vi "Configure Trigger Synchronization.vi"(0 "niUsrpRio Session":T1={"Global Settings Register Bus"=refnum, "Radio 0 Settings Register Bus"=refnum, "Rx NI-USRP session"="", "Tx NI-USRP session"="", "FPGA Interface"=refnum, "RIO Interface Number"=0, "EEPROM Header"={"Checksum"=0, "Product Code"=0, "Hardware Current Version"=0, "Hardware Oldest Compatible Version"=0, "EEPROM Map Current Version"=0, "EEPROM Map Oldest Compatible Version"=0, "User Password"="", "Pointer to Factory Header"=0, "Pointer to User Header"=0, "Recommended Interval"=0, "Number of Reserved Bytes"=9, "Number of Daughterboards"=0, "Daughterboard IDs"=[], "Daughterboard Serial Numbers"=[]}, "Device Data Header"={"Checksum"=0, "Number of Channels"=0, "Number of Gain Settings"=[], "Pointer to Characterization Data"=[], "Number of Reserved Bytes"=27, "Number of Frequencies"=[]}, "EEPROM Characterization Header"={"Checksum"=0, "Date"=timestamp(0 s since 1904-01-01), "Temperature"=0.0, "Misc. Info"="", "Pointer to Device Data Header"=0, "Number of Reserved Bytes"=28}, "Characterization Data"=[], "Characterization Data Valid?"=FALSE, "Radio 1 Settings Register Bus"=refnum, "Radio Settings Bus Semaphore"=refnum} {"Characterization Data"."Frequencies [Hz]" format="%#_6p"; "EEPROM Characterization Header"."Pointer to Device Data Header" format="%x"; "EEPROM Characterization Header"."Checksum" format="%x"; "Device Data Header"."Pointer to Characterization Data" format="%x"; "Device Data Header"."Checksum" format="%x"; "EEPROM Header"."Pointer to User Header" format="%x"; "EEPROM Header"."Pointer to Factory Header" format="%x"; "EEPROM Header"."Product Code" format="%x"; "EEPROM Header"."Checksum" format="%x"}, 1 "scope":string(combo)="rx", 5 "enable trigger synchronization":bool, 11 "error in":errorcluster) -> (4 "niUsrpRio Session (out)":T1={"Global Settings Register Bus"=refnum, "Radio 0 Settings Register Bus"=refnum, "Rx NI-USRP session"="", "Tx NI-USRP session"="", "FPGA Interface"=refnum, "RIO Interface Number"=0, "EEPROM Header"={"Checksum"=0, "Product Code"=0, "Hardware Current Version"=0, "Hardware Oldest Compatible Version"=0, "EEPROM Map Current Version"=0, "EEPROM Map Oldest Compatible Version"=0, "User Password"="", "Pointer to Factory Header"=0, "Pointer to User Header"=0, "Recommended Interval"=0, "Number of Reserved Bytes"=9, "Number of Daughterboards"=0, "Daughterboard IDs"=[], "Daughterboard Serial Numbers"=[]}, "Device Data Header"={"Checksum"=0, "Number of Channels"=0, "Number of Gain Settings"=[], "Pointer to Characterization Data"=[], "Number of Reserved Bytes"=27, "Number of Frequencies"=[]}, "EEPROM Characterization Header"={"Checksum"=0, "Date"=timestamp(0 s since 1904-01-01), "Temperature"=0.0, "Misc. Info"="", "Pointer to Device Data Header"=0, "Number of Reserved Bytes"=28}, "Characterization Data"=[], "Characterization Data Valid?"=FALSE, "Radio 1 Settings Register Bus"=refnum, "Radio Settings Bus Semaphore"=refnum} {"Characterization Data"."Frequencies [Hz]" format="%#_6p"; "EEPROM Characterization Header"."Pointer to Device Data Header" format="%x"; "EEPROM Characterization Header"."Checksum" format="%x"; "Device Data Header"."Pointer to Characterization Data" format="%x"; "Device Data Header"."Checksum" format="%x"; "EEPROM Header"."Pointer to User Header" format="%x"; "EEPROM Header"."Pointer to Factory Header" format="%x"; "EEPROM Header"."Product Code" format="%x"; "EEPROM Header"."Checksum" format="%x"}, 15 "error out":errorcluster)   [LabVIEW 2013]
doc: "Enables or disables trigger synchronization. Trigger synchronization is controlled by the FPGA, and must be configured before sending a start trigger."
uses:
  <instrlib>/niUsrpRio/Config/v1/Host/Public/niUsrpRio Session.ctl
  <instrlib>/_niInstr/Register Bus/v0/Host/Public/Register Bus Session.ctl
  <instrlib>/_niInstr/Register Bus/v0/Host/Private/Session Data.ctl
  <instrlib>/niUsrpRio/Config/v1/Host/Public/EEPROM Header.ctl
  <instrlib>/niUsrpRio/Config/v1/Host/Public/EEPROM Device Data Header.ctl
  <instrlib>/niUsrpRio/Config/v1/Host/Public/EEPROM Characterization Header.ctl
  <instrlib>/niUsrpRio/Config/v1/Host/Public/Characterization Data.ctl
  <instrlib>/niUsrpRio/Config/v1/Host/Public/IQ Imbalance.ctl
  Rx FPGA VI Reference.ctl
  Tx FPGA VI Reference.ctl
  <vilib>/rvi/interface/common/niFpgaWaitOnOcc.vi
  <vilib>/Utility/error.llb/Error Cluster From Error Code.vi
  <vilib>/rvi/errors/niLvFpgaAdjustHostInterfaceError.vi
  <vilib>/rvi/interface/nirviReadWriteControl/nirviReadWriteControl.xnode
  NiFpgaLv.dll
  <vilib>/rvi/interface/Simulation/niFpgaSimulationCallBeginRW.vi
  <instrlib>/niUsrpRio/Config/v1/Host/niUsrpRio Config v1 Host.lvlib
  <instrlib>/_niInstr/Register Bus/v0/Host/niInstr Register Bus v0 Host.lvlib
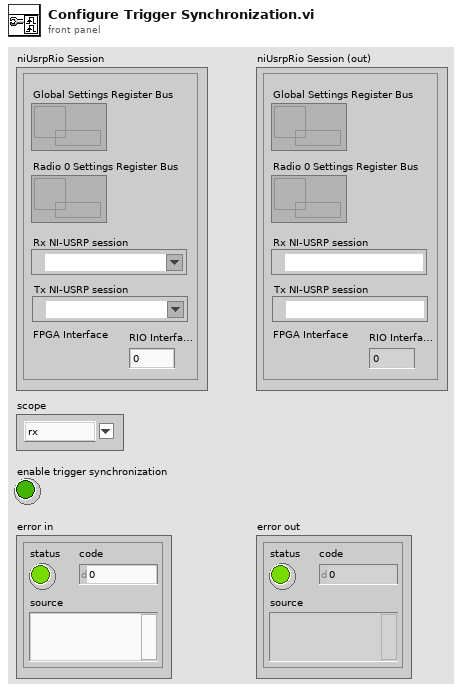
[diagram p1: front panel]
types:
  T1 = typedef "niUsrpRio Config v1 Host.lvlib/niUsrpRio Session.ctl" = cluster{"Global Settings Register Bus":T2, "Radio 0 Settings Register Bus":T2, "Rx NI-USRP session":refnum<k15>, "Tx NI-USRP session":refnum<k15>, "FPGA Interface":refnum<k20>, "RIO Interface Number":u32, "EEPROM Header":T3, "Device Data Header":T4, "EEPROM Characterization Header":T5, "Characterization Data":T6[], "Characterization Data Valid?":bool, "Radio 1 Settings Register Bus":T2, "Radio Settings Bus Semaphore":T8}
  T2 = typedef "niInstr Register Bus v0 Host.lvlib/Register Bus Session.ctl" = refnum<queue>
  T3 = typedef "niUsrpRio Config v1 Host.lvlib/EEPROM Header.ctl" = cluster{"Checksum":u32, "Product Code":u16, "Hardware Current Version":u16, "Hardware Oldest Compatible Version":u16, "EEPROM Map Current Version":u16, "EEPROM Map Oldest Compatible Version":u16, "User Password":string, "Pointer to Factory Header":u32, "Pointer to User Header":u32, "Recommended Interval":u16, "Number of Reserved Bytes":i32, "Number of Daughterboards":u8, "Daughterboard IDs":u16[], "Daughterboard Serial Numbers":string[]}
  T4 = typedef "niUsrpRio Config v1 Host.lvlib/EEPROM Device Data Header.ctl" = cluster{"Checksum":u32, "Number of Channels":u8, "Number of Gain Settings":u16[], "Pointer to Characterization Data":u32[], "Number of Reserved Bytes":i32, "Number of Frequencies":u16[]}
  T5 = typedef "niUsrpRio Config v1 Host.lvlib/EEPROM Characterization Header.ctl" = cluster{"Checksum":u32, "Date":timestamp, "Temperature":sgl, "Misc. Info":string, "Pointer to Device Data Header":u32, "Number of Reserved Bytes":i32}
  T6 = typedef "niUsrpRio Config v1 Host.lvlib/Characterization Data.ctl" = cluster{"Gains[dB]":dbl[], "Frequencies [Hz]":dbl[], "IQ Imbalance Table":T7[], "Measured Gains[dB]":dbl[][]}
  T7 = typedef "niUsrpRio Config v1 Host.lvlib/IQ Imbalance.ctl" = cluster{"Gain Imbalance [linear]":dbl, "Phase Imbalance [radians]":dbl, "Offset":cdb}
  T8 = typedef "Semaphore RefNum" = refnum<k1>
  T9 = typedef "niUsrpRio Config v1 Host.lvlib/Device Subfunction.ctl" = enum16{"rx", "tx"}
  T10 = typedef "Rx FPGA VI Reference.ctl" = refnum<k20>
  T11 = typedef "Tx FPGA VI Reference.ctl" = refnum<k20>
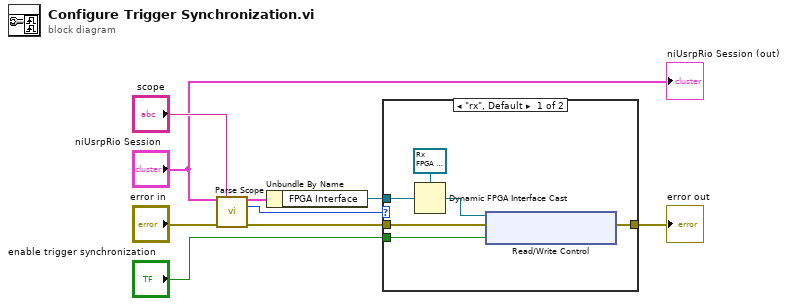
[diagram p0: block diagram]
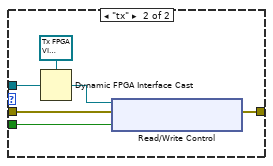
[diagram p2: hidden frame]
diagram:
  n1 = call <instrlib>:"Parse Scope.vi"("niUsrpRio Session"="niUsrpRio Session", "scope"="scope", "Error In"="error in") -> ("niUsrpRio Session (out)"=w4:T1, "Device Subfunction"=w3:T9, "Error Out"=w5:errorcluster)  [unwired: 4 in, 6 out]
  n2 = Unbundle By Name(w4) -> ("FPGA Interface"=w6:refnum<k20>)
  n3 = case shown="\"rx\", Default" w3 {
    tunnel: w5 -> [w15 w21]
    tunnel: w6 -> [w14 w20]
    tunnel: [w12 w18] -> w7
    tunnel: "enable trigger synchronization" -> [w10 w16]
    frame "rx", Default {
      n4 = Dynamic FPGA Interface Cast(Session In=T10 refnum ("Rx FPGA VI Reference"), Type=w14) -> (Session Out=w13:T10)
      n5 = xnode "Read/Write Control"("FPGA VI Reference In"=w13, "error in"=w15, "rx.enable trigger sync"=w10) -> ("error out"=w12:errorcluster)  [unwired: 1 out]
    }
    frame "tx" {
      n6 = Dynamic FPGA Interface Cast(Session In=T11 refnum ("Tx FPGA VI Reference"), Type=w20) -> (Session Out=w19:T11)
      n7 = xnode "Read/Write Control"("FPGA VI Reference In"=w19, "error in"=w21, "tx.enable trigger sync"=w16) -> ("error out"=w18:errorcluster)  [unwired: 1 out]
    }
  }
  "error out" <- w7
  "niUsrpRio Session (out)" <- "niUsrpRio Session"
